vi "DT.vi"(9 "output option":T1 items=["Triangle", "Adj Triangle", "Segment"], 10 "Y":dbl[](array[numeric]), 11 "X":dbl[](array[numeric])) -> (0 "error":i32, 3 "Triangles":i32[][](array[numeric]))   [LabVIEW 2017, in "NI_AAL_Geometry.lvlib"]
uses:
  <vilib>/Analysis/NI_AAL_Geometry.lvlib
  <vilib>/Analysis/geometry.llb/DT_Output Option.ctl
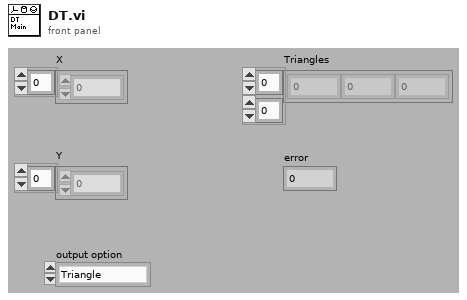
[diagram p1: front panel]
types:
  T1 = typedef "NI_AAL_Geometry.lvlib/DT_Output Option.ctl" = i32
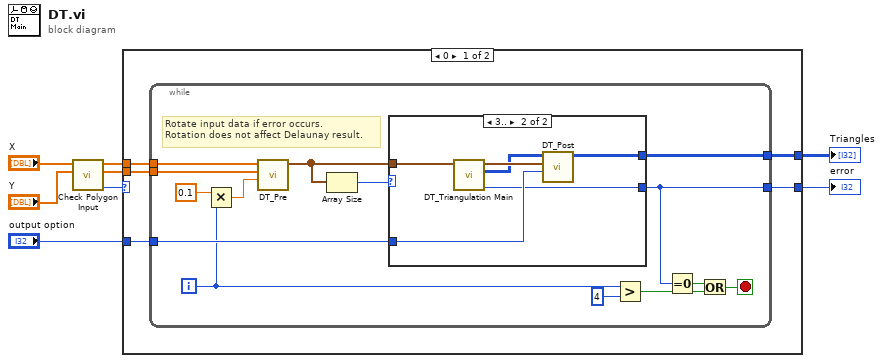
[diagram p0: block diagram]
diagram:
  n1 = call <vilib>:"Check Polygon Input.vi"("Y In"="Y", "X In"="X") -> ("error"=w6:i32, "Y Out"=w4:dbl[], "X Out"=w5:dbl[])  [unwired: 7 in]
  n2 = case shown="0" w6 {
    selector: w6 -> [_ w34]
    tunnel: w5 -> [w13 _]
    tunnel: w4 -> [w12 _]
    tunnel: [w9 w34] -> w3
    tunnel: [w11 _] -> w2
    tunnel: "output option" -> [w10 _]
    frame 0 {
      n3 = while {
        tunnel: w13 -> [w27]
        tunnel: w12 -> [w26]
        tunnel: [w25] -> w11
        tunnel: w10 -> [w22]
        tunnel: [w19] -> w9
        i -> [w18]
        stop <- w14 stop-if-true
        # "Rotate input data if error occurs.\nRotation does not affect Delaunay result."
        n4 = Multiply(x=0.1, y=w18) -> (x*y=w20:dbl)
        n5 = call <vilib>:"DT_Pre.vi"("rotation angle"=w20, "Y"=w26, "X"=w27) -> ("Points"=w23:cluster{"x":dbl, "y":dbl, "index":i32}[])  [unwired: 8 out]
        n6 = Array Size(array=w23) -> (size(s)=w24:i32)
        n7 = case shown="3.." w24 {
          tunnel: [_ w33] -> w25
          tunnel: w23 -> [_ w32]
          tunnel: w22 -> [_ w29]
          tunnel: [_ w28] -> w19
          frame 0, Default {
            # "Number of distinct points is less than 3.\nNo triangles can be found."
          }
          frame 3.. {
            n8 = call <vilib>:"DT_Triangulation Main.vi"("Points In"=w32) -> ("error"=w28:i32, "Triangles"=w30:i32[][], "Points Out"=w31:cluster{"x":dbl, "y":dbl, "index":i32}[])  [unwired: 8 out]
            n9 = call <vilib>:"DT_Post.vi"("output option"=w29, "Points"=w31, "Triangles In"=w30) -> ("Triangles Out"=w33:i32[][])  [unwired: 8 out]
          }
        }
        n10 = Greater?(x=w18, y=4) -> (0:w16:bool)
        n11 = Equal To 0?(x=w19) -> (x = 0?=w15:bool)
        n12 = Or(x=w15, y=w16) -> (x .or. y?=w14:bool)
      }
    }
    frame -1, Default {
    }
  }
  "Triangles" <- w2
  "error" <- w3
